vi "3030-HS - DAC.VI"() -> ()   [LabVIEW 2015]
uses:
  board.vis/Globals.vi
  <vilib>/Analysis/NI_AALBase.lvlib
panel:
  in  "extTrig":bool
  in  "ext. trig. slope":enum32{"1", "2", "3"}(radio)
  in  "send all":bool
  in  "Offset ADC 8":u16=49000
  in  "Offset ADC 3":u16=49000
  in  "Offset ADC 7":u16=49000
  in  "Offset ADC 2":u16=49000
  in  "Offset ADC 6":u16=49000
  in  "Offset ADC 1":u16=49000
  in  "Offset ADC 5":u16=49000
  in  "Offset ADC 4":u16=49000
  out "tRMS":dbl=11.563017373787728 format="%0#.1f"
  out "mean":dbl=8306.733333333334 format="%#_4f"
  in  "rms_pixel":u16=100
  in  "continuous":bool
  out "curr.block":u8=1
  out "Measure ON":bool
  in  "Board select\n1: board 1\n2: board 2\n3: both boards":u8=3
  in  "no.of blocks (nob)\npress enter":u32=1
  in  "block":u32(slide)=1 max=10 scale=0.9..1.0
  out "Signalverlaufgraph 2":u16[](graph)=[0, 0, 543, 543, 0, 1, 0, 0, 2, 2, 3, 3, 4, 4, 5, 5, 6, 6, 7, 7, 8, 8, 9, 9, 10, 10, 11, 11, 12, 12, 13, 13, 14, 14, 15, 15, 16, 16, 17, 17, 18, 18, 19, 19, 20, 20, 21, 21, 22, 22, 23, 23, 24, 24, 25, 25, 26, 26, 27, 27, 28, 28, 29, 29, 30, 30, 31, 31, 32, 32, 33, 33, 34, 34, 35, 35, 36, 36, 37, 37, 38, 38, 39, 39, 40, 40, 41, 41, 42, 42, 43, 43, 44, 44, 45, 45, 46, 46, 47, 47, 48, 48, 49, 49, 50, 50, 51, 51, 52, 52, 53, 53, 54, 54, 55, 55, 56, 56, 57, 57, 58, 58, 59, 59, 60, 60, 61, 61, 62, 62, 63, 63, 64, 64, 65, 65, 66, 66, 67, 67, 68, 68, 69, 69, 70, 70, 71, 71, 72, 72, 73, 73, 74, 74, 75, 75, 76, 76, 77, 77, 78, 78, 79, 79, 80, 80, 81, 81, 82, 82, 83, 83, 84, 84, 85, 85, 86, 86, 87, 87, 88, 88, 89, 89, 90, 90, 91, 91, 92, 92, 93, 93, 94, 94, 95, 95, 96, 96, 97, 97, 98, 98, 99, 99, 100, 100, 101, 101, 102, 102, 103, 103, 104, 104, 105, 105, 106, 106, 107, 107, 108, 108, 109, 109, 110, 110, 111, 111, 112, 112, 113, 113, 114, 114, 115, 115, 116, 116, 117, 117, 118, 118, 119, 119, 120, 120, 121, 121, 122, 122, 123, 123, 124, 124, 125, 125, 126, 126, 127, 127, 128, 128, 129, 129, 130, 130, 131, 131, 132, 132, 133, 133, 134, 134, 135, 135, 136, 136, 137, 137, 138, 138, 139, 139, 140, 140, 141, 141, 142, 142, 143, 143, 144, 144, 145, 145, 146, 146, 147, 147, 148, 148, 149, 149, 150, 150, 151, 151, 152, 152, 153, 153, 154, 154, 155, 155, 156, 156, 157, 157, 158, 158, 159, 159, 160, 160, 161, 161, 162, 162, 163, 163, 164, 164, 165, 165, 166, 166, 167, 167, 168, 168, 169, 169, 170, 170, 171, 171, 172, 172, 173, 173, 174, 174, 175, 175, 176, 176, 177, 177, 178, 178, 179, 179, 180, 180, 181, 181, 182, 182, 183, 183, 184, 184, 185, 185, 186, 186, 187, 187, 188, 188, 189, 189, 190, 190, 191, 191, 192, 192, 193, 193, 194, 194, 195, 195, 196, 196, 197, 197, 198, 198, 199, 199, 200, 200, 201, 201, 202, 202, 203, 203, 204, 204, 205, 205, 206, 206, 207, 207, 208, 208, 209, 209, 210, 210, 211, 211, 212, 212, 213, 213, 214, 214, 215, 215, 216, 216, 217, 217, 218, 218, 219, 219, 220, 220, 221, 221, 222, 222, 223, 223, 224, 224, 225, 225, 226, 226, 227, 227, 228, 228, 229, 229, 230, 230, 231, 231, 232, 232, 233, 233, 234, 234, 235, 235, 236, 236, 237, 237, 238, 238, 239, 239, 240, 240, 241, 241, 242, 242, 243, 243, 244, 244, 245, 245, 246, 246, 247, 247, 248, 248, 249, 249, 250, 250, 251, 251, 252, 252, 253, 253, 254, 254, 255, 255, 256, 256, 257, 257, 258, 258, 259, 259, 260, 260, 261, 261, 262, 262, 263, 263, 264, 264, 265, 265, 266, 266, 267, 267, 268, 268, 269, 269, 270, 270, 271, 271, 272, 272, 273, 273, 274, 274, 275, 275, 276, 276, 277, 277, 278, 278, 279, 279, 280, 280, 281, 281, 282, 282, 283, 283, 284, 284, 285, 285, 286, 286, 287, 287, 288, 288, 289, 289, 290, 290, 291, 291, 292, 292, 293, 293, 294, 294, 295, 295, 296, 296, 297, 297, 298, 298, 299, 299, 300, 300, 301, 301, 302, 302, 303, 303, 304, 304, 305, 305, 306, 306, 307, 307, 308, 308, 309, 309, 310, 310, 311, 311, 312, 312, 313, 313, 314, 314, 315, 315, 316, 316, 317, 317, 318, 318, 319, 319, 320, 320, 321, 321, 322, 322, 323, 323, 324, 324, 325, 325, 326, 326, 327, 327, 328, 328, 329, 329, 330, 330, 331, 331, 332, 332, 333, 333, 334, 334, 335, 335, 336, 336, 337, 337, 338, 338, 339, 339, 340, 340, 341, 341, 342, 342, 343, 343, 344, 344, 345, 345, 346, 346, 347, 347, 348, 348, 349, 349, 350, 350, 351, 351, 352, 352, 353, 353, 354, 354, 355, 355, 356, 356, 357, 357, 358, 358, 359, 359, 360, 360, 361, 361, 362, 362, 363, 363, 364, 364, 365, 365, 366, 366, 367, 367, 368, 368, 369, 369, 370, 370, 371, 371, 372, 372, 373, 373, 374, 374, 375, 375, 376, 376, 377, 377, 378, 378, 379, 379, 380, 380, 381, 381, 382, 382, 383, 383, 384, 384, 385, 385, 386, 386, 387, 387, 388, 388, 389, 389, 390, 390, 391, 391, 392, 392, 393, 393, 394, 394, 395, 395, 396, 396, 397, 397, 398, 398, 399, 399, 400, 400, 401, 401, 402, 402, 403, 403, 404, 404, 405, 405, 406, 406, 407, 407, 408, 408, 409, 409, 410, 410, 411, 411, 412, 412, 413, 413, 414, 414, 415, 415, 416, 416, 417, 417, 418, 418, 419, 419, 420, 420, 421, 421, 422, 422, 423, 423, 424, 424, 425, 425, 426, 426, 427, 427, 428, 428, 429, 429, 430, 430, 431, 431, 432, 432, 433, 433, 434, 434, 435, 435, 436, 436, 437, 437, 438, 438, 439, 439, 440, 440, 441, 441, 442, 442, 443, 443, 444, 444, 445, 445, 446, 446, 447, 447, 448, 448, 449, 449, 450, 450, 451, 451, 452, 452, 453, 453, 454, 454, 455, 455, 456, 456, 457, 457, 458, 458, 459, 459, 460, 460, 461, 461, 462, 462, 463, 463, 464, 464, 465, 465, 466, 466, 467, 467, 468, 468, 469, 469, 470, 470, 471, 471, 472, 472, 473, 473, 474, 474, 475, 475, 476, 476, 477, 477, 478, 478, 479, 479, 480, 480, 481, 481, 482, 482, 483, 483, 484, 484, 485, 485, 486, 486, 487, 487, 488, 488, 489, 489, 490, 490, 491, 491, 492, 492, 493, 493, 494, 494, 495, 495, 496, 496, 497, 497, 498, 498, 499, 499, 500, 500, 501, 501, 502, 502, 503, 503, 504, 504, 505, 505, 506, 506, 507, 507, 508, 508, 509, 509, 510, 510, 511, 511, 512, 512, 513, 513, 514, 514, 515, 515, 516, 516, 517, 517, 518, 518, 519, 519, 520, 520, 521, 521, 522, 522, 523, 523, 524, 524, 525, 525, 526, 526, 527, 527, 528, 528, 529, 529, 530, 530, 531, 531, 532, 532, 533, 533, 534, 534, 535, 535, 536, 536, 537, 537, 538, 538, 539, 539, 540, 540, 541, 541]
  out "Signalverlaufgraph":u16[](graph)=[8087, 8087, 8087, 8087, 49152, 1, 0, 50, 7170, 7170, 7521, 7730, 7840, 7916, 7976, 8049, 8112, 8160, 8204, 8214, 8236, 8264, 8286, 8290, 8324, 8328, 8343, 8353, 8359, 8375, 8388, 8394, 8403, 8403, 8394, 8394, 8388, 8378, 8378, 8372, 8362, 8347, 8340, 8334, 8331, 8343, 8340, 8331, 8321, 8312, 8309, 8312, 8302, 8315, 8321, 8324, 8328, 8312, 8309, 8299, 8312, 8305, 8309, 8293, 8318, 8309, 8305, 8315, 8321, 8318, 8312, 8305, 8312, 8290, 8302, 8274, 8280, 8290, 8305, 8305, 8299, 8324, 8305, 8302, 8302, 8302, 8312, 8309, 8315, 8309, 8296, 8296, 8299, 8305, 8312, 8309, 8299, 8302, 8305, 8296, 8305, 8299, 8299, 8296, 8293, 8302, 8280, 8290, 8302, 8305, 8286, 8283, 8283, 8280, 8293, 8290, 8290, 8274, 8280, 8271, 8252, 8258, 8245, 8255, 8248, 8258, 8264, 8271, 8286, 8283, 8277, 8280, 8274, 8264, 8258, 8261, 8255, 8255, 7094, 7258, 7407, 7568, 7742, 7900, 8005, 8103, 8135, 8157, 8198, 8207, 8245, 8252, 8264, 8271, 8286, 8296, 8318, 8343, 8340, 8343, 8334, 8334, 8315, 8340, 8334, 8328, 8324, 8318, 8309, 8302, 8290, 8286, 8290, 8283, 8267, 8255, 8264, 8255, 8252, 8255, 8242, 8264, 8258, 8258, 8248, 8248, 8264, 8236, 8229, 8255, 8248, 8245, 8255, 8267, 8258, 8248, 8264, 8248, 8236, 8226, 8217, 8245, 8226, 8233, 8236, 8239, 8252, 8252, 8261, 8245, 8267, 8258, 8258, 8258, 8252, 8255, 8258, 8239, 8239, 8242, 8239, 8239, 8226, 8236, 8233, 8239, 8214, 8226, 8223, 8226, 8226, 8242, 8229, 8229, 8242, 8229, 8233, 8220, 8226, 8220, 8226, 8226, 8229, 8229, 8226, 8201, 8198, 8207, 8204, 8192, 8192, 8201, 8220, 8229, 8214, 8214, 8226, 8229, 8233, 8214, 8214, 8198, 8201, 8198, 8201, 8201, 7535, 7706, 7869, 8014, 8163, 8298, 8426, 8504, 8546, 8599, 8642, 8670, 8685, 8716, 8734, 8738, 8745, 8777, 8787, 8816, 8833, 8833, 8841, 8855, 8830, 8833, 8823, 8816, 8805, 8805, 8798, 8787, 8787, 8773, 8791, 8787, 8777, 8773, 8773, 8766, 8759, 8759, 8763, 8763, 8766, 8763, 8752, 8755, 8741, 8748, 8745, 8734, 8741, 8755, 8763, 8763, 8763, 8755, 8745, 8745, 8734, 8755, 8745, 8748, 8724, 8724, 8731, 8745, 8741, 8741, 8745, 8731, 8738, 8741, 8738, 8741, 8731, 8745, 8748, 8748, 8731, 8731, 8727, 8713, 8720, 8731, 8727, 8731, 8720, 8724, 8724, 8731, 8716, 8731, 8734, 8731, 8741, 8734, 8724, 8716, 8709, 8724, 8720, 8709, 8713, 8706, 8713, 8695, 8706, 8695, 8692, 8688, 8685, 8688, 8685, 8706, 8695, 8699, 8709, 8702, 8702, 8706, 8702, 8692, 8699, 8695, 8688, 8688, 7100, 7287, 7448, 7622, 7783, 7942, 8049, 8125, 8160, 8204, 8233, 8239, 8271, 8283, 8286, 8302, 8312, 8312, 8328, 8350, 8359, 8381, 8356, 8350, 8350, 8350, 8334, 8321, 8328, 8334, 8318, 8321, 8309, 8296, 8293, 8293, 8305, 8286, 8277, 8280, 8277, 8283, 8280, 8283, 8290, 8280, 8274, 8264, 8258, 8277, 8258, 8274, 8271, 8280, 8283, 8302, 8283, 8290, 8293, 8280, 8258, 8274, 8264, 8271, 8271, 8271, 8271, 8290, 8277, 8267, 8283, 8267, 8267, 8264, 8286, 8283, 8280, 8290, 8286, 8290, 8283, 8274, 8290, 8271, 8277, 8274, 8286, 8274, 8261, 8261, 8261, 8267, 8274, 8274, 8274, 8283, 8280, 8261, 8264, 8267, 8261, 8258, 8258, 8248, 8248, 8245, 8239, 8236, 8226, 8233, 8239, 8223, 8223, 8226, 8245, 8239, 8245, 8255, 8245, 8255, 8255, 8236, 8245, 8236, 8239, 8229, 8245, 8245, 7777, 7964, 8135, 8271, 8435, 8546, 8647, 8717, 8783, 8834, 8856, 8872, 8878, 8888, 8900, 8922, 8919, 8938, 8954, 8967, 8979, 8992, 8986, 8992, 8967, 8986, 8964, 8957, 8941, 8945, 8941, 8941, 8941, 8932, 8935, 8922, 8926, 8926, 8926, 8922, 8919, 8907, 8910, 8919, 8907, 8922, 8913, 8919, 8907, 8900, 8903, 8897, 8903, 8903, 8922, 8919, 8922, 8913, 8916, 8910, 8903, 8891, 8888, 8891, 8869, 8891, 8891, 8907, 8910, 8888, 8903, 8916, 8900, 8903, 8916, 8910, 8913, 8897, 8913, 8894, 8897, 8897, 8884, 8894, 8888, 8891, 8891, 8891, 8894, 8884, 8884, 8888, 8878, 8884, 8897, 8888, 8881, 8888, 8884, 8897, 8875, 8884, 8881, 8894, 8891, 8884, 8865, 8853, 8853, 8850, 8862, 8840, 8853, 8853, 8869, 8859, 8853, 8865, 8872, 8894, 8881, 8862, 8856, 8853, 8853, 8865, 8862, 8862, 7511, 7713, 7894, 8089, 8284, 8458, 8603, 8702, 8773, 8794, 8830, 8851, 8865, 8876, 8890, 8873, 8894, 8915, 8919, 8968, 8982, 8968, 8979, 8968, 8954, 8968, 8940, 8936, 8940, 8929, 8922, 8929, 8901, 8901, 8915, 8912, 8897, 8912, 8897, 8897, 8887, 8876, 8873, 8869, 8897, 8897, 8883, 8883, 8862, 8876, 8851, 8869, 8876, 8876, 8894, 8897, 8876, 8890, 8883, 8880, 8851, 8858, 8841, 8841, 8830, 8844, 8862, 8880, 8873, 8876, 8887, 8883, 8876, 8887, 8890, 8890, 8887, 8897, 8901, 8890, 8876, 8851, 8883, 8862, 8851, 8873, 8876, 8869, 8855, 8862, 8851, 8855, 8851, 8858, 8876, 8869, 8865, 8869, 8858, 8865, 8862, 8873, 8844, 8862, 8858, 8869, 8855, 8844, 8837, 8841, 8837, 8826, 8823, 8837, 8848, 8862, 8844, 8865, 8862, 8855, 8862, 8844, 8830, 8830, 8826, 8830, 8844, 8844, 8071, 8252, 8397, 8555, 8714, 8853, 8960, 9027, 9071, 9115, 9138, 9150, 9191, 9195, 9210, 9204, 9217, 9229, 9245, 9264, 9293, 9280, 9283, 9277, 9264, 9277, 9248, 9245, 9242, 9232, 9229, 9229, 9236, 9210, 9223, 9220, 9226, 9204, 9195, 9201, 9195, 9204, 9191, 9188, 9207, 9204, 9198, 9204, 9195, 9176, 9188, 9176, 9179, 9198, 9188, 9182, 9179, 9198, 9195, 9188, 9179, 9179, 9166, 9169, 9163, 9157, 9172, 9188, 9179, 9191, 9188, 9182, 9188, 9201, 9188, 9198, 9179, 9188, 9191, 9188, 9179, 9188, 9176, 9182, 9179, 9185, 9182, 9179, 9169, 9157, 9163, 9169, 9172, 9182, 9201, 9191, 9185, 9188, 9182, 9169, 9172, 9172, 9163, 9176, 9179, 9169, 9153, 9157, 9141, 9150, 9147, 9131, 9122, 9160, 9153, 9160, 9160, 9153, 9160, 9163, 9157, 9157, 9134, 9138, 9147, 9125, 9144, 9144, 7606, 7787, 7957, 8122, 8299, 8432, 8543, 8603, 8657, 8682, 8720, 8742, 8761, 8767, 8780, 8783, 8796, 8799, 8808, 8818, 8837, 8843, 8853, 8834, 8827, 8837, 8812, 8802, 8802, 8799, 8780, 8790, 8767, 8771, 8796, 8790, 8771, 8767, 8764, 8764, 8752, 8742, 8755, 8764, 8767, 8783, 8755, 8752, 8739, 8742, 8755, 8739, 8748, 8736, 8761, 8764, 8758, 8767, 8758, 8761, 8742, 8736, 8736, 8736, 8698, 8704, 8736, 8736, 8748, 8748, 8764, 8761, 8755, 8758, 8745, 8748, 8755, 8758, 8755, 8758, 8739, 8736, 8723, 8729, 8726, 8736, 8736, 8739, 8733, 8717, 8714, 8720, 8710, 8729, 8752, 8742, 8745, 8739, 8739, 8742, 8726, 8733, 8742, 8739, 8736, 8729, 8707, 8707, 8704, 8717, 8704, 8695, 8688, 8695, 8723, 8729, 8720, 8717, 8720, 8739, 8733, 8707, 8710, 8710, 8704, 8717, 8742, 8742, 8264, 8226, 8188, 8141, 8097, 8097, 8097, 8097, 8097, 8097, 8097, 8097, 8097, 8097, 8097, 8097, 8097, 8097, 8097, 8097, 8097, 8097, 8097, 8097, 8097, 8097, 8097, 8097, 8097, 8097, 8097, 8097, 8097, 8097, 8097, 8097, 8097, 8097, 8097, 8097, 8097, 8097, 8097, 8097, 8097, 8097, 8097, 8097, 8097, 8097, 8097, 8097, 8097, 8097]
  out "boards recognised":u8=2
  in  "alloc mem":bool
  out "FREE \nRAM MB":dbl=13718.2421875
  out "BUILT-IN\nRAM MB":dbl=16271.7421875
  out "SEC":dbl=0.01
  out "MB RAM":dbl=0.20751953125
  in  "DAT in 10ns":u32
  in  "stop all":bool
  in  "start":bool
  in  "sample":u32(slide)=51 max=3000 scale=0.9..100.0
  in  "no.of samples (nos)":u32=1000
  in  "exposuretime[ms]":dbl=0.04 format="%.3f"
  # "press Esc to stop\nmeasurement"
  # "exit here"
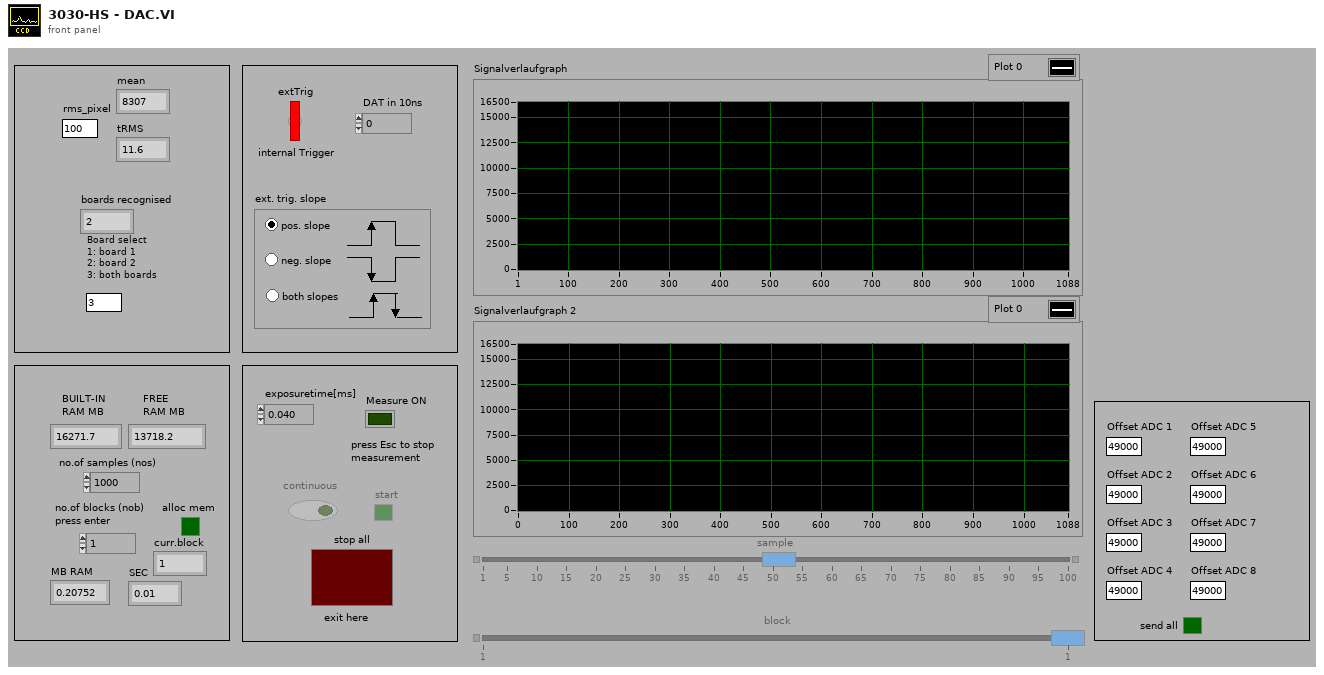
[diagram p1: front panel]
types:
  T1 = enum8{"Enabled", "Disabled", "Disabled and Grayed Out"}
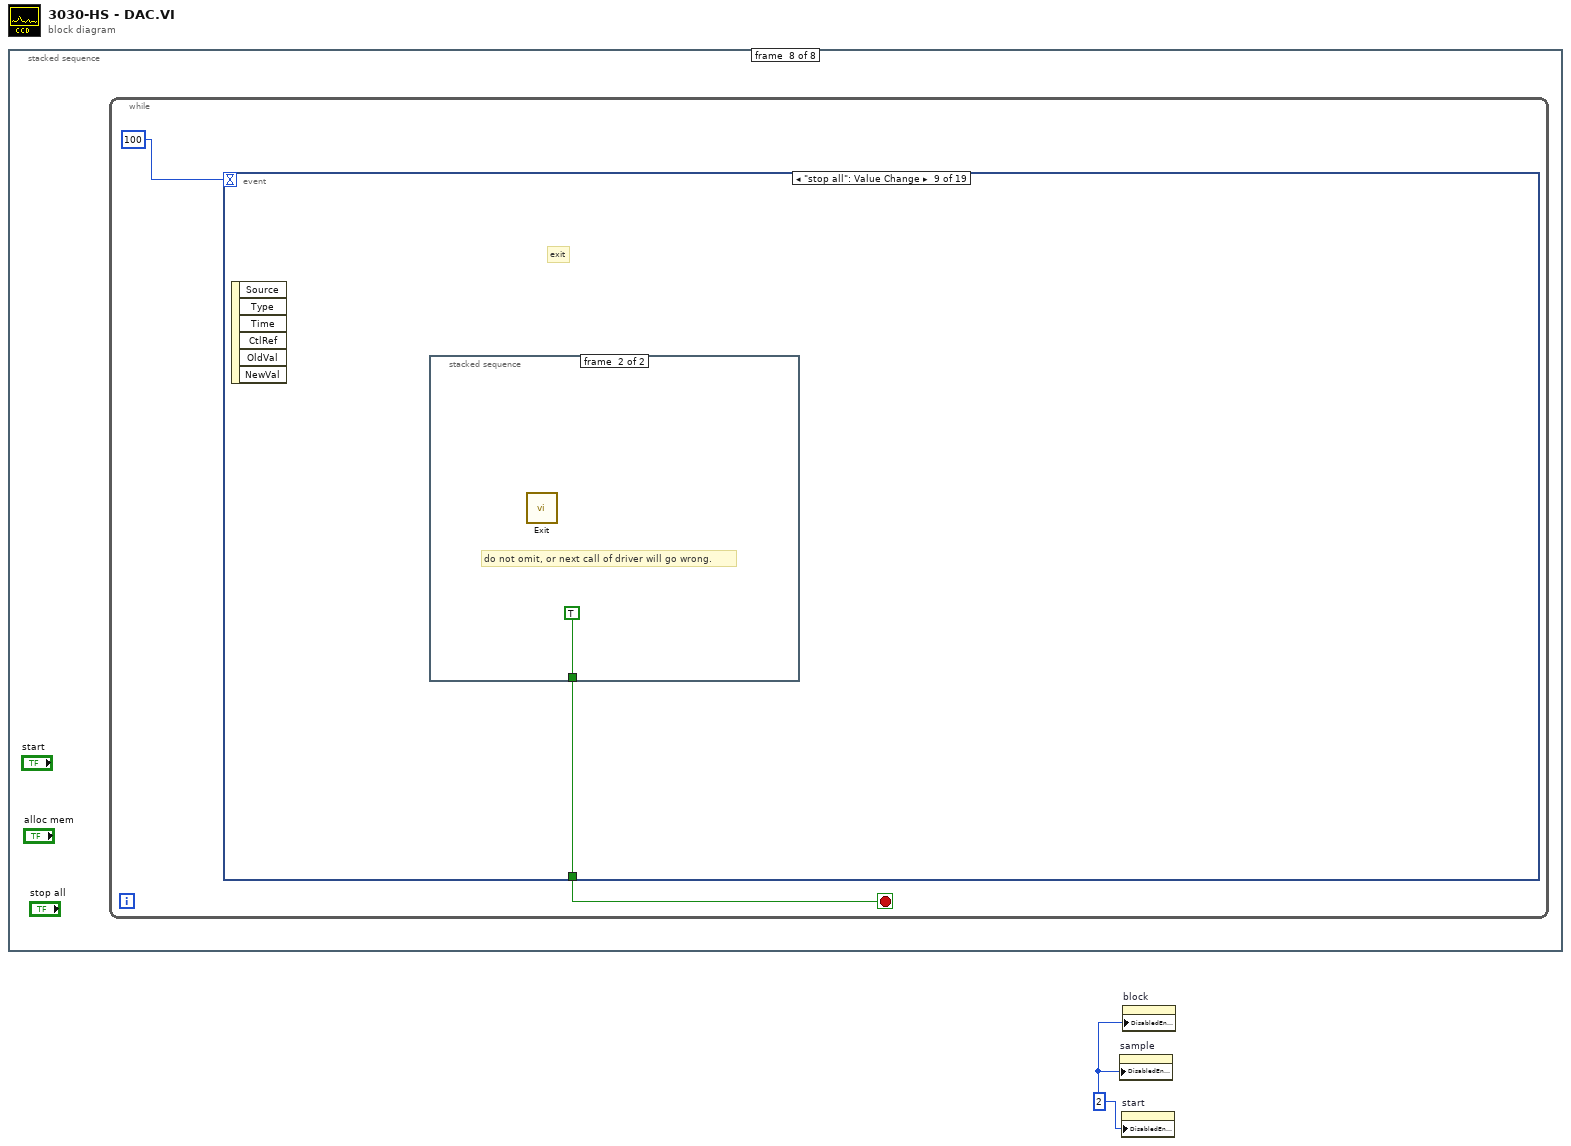
[diagram p0: block diagram]
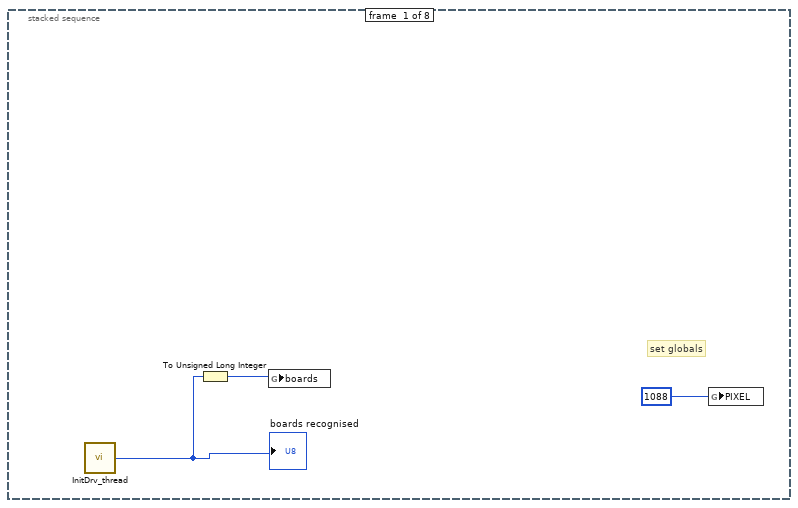
[diagram p2: hidden frame]
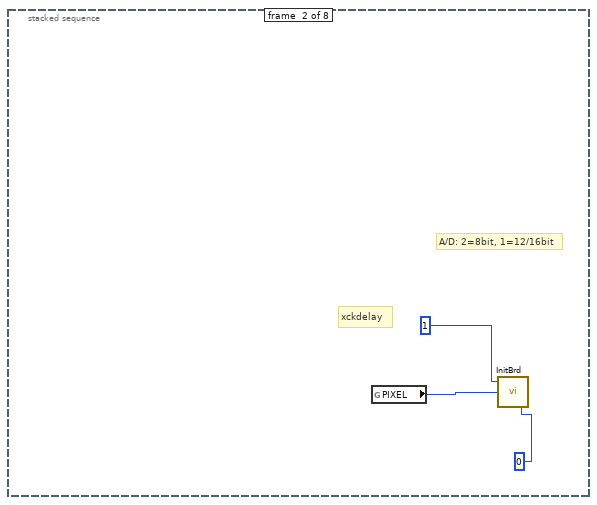
[diagram p3: hidden frame]
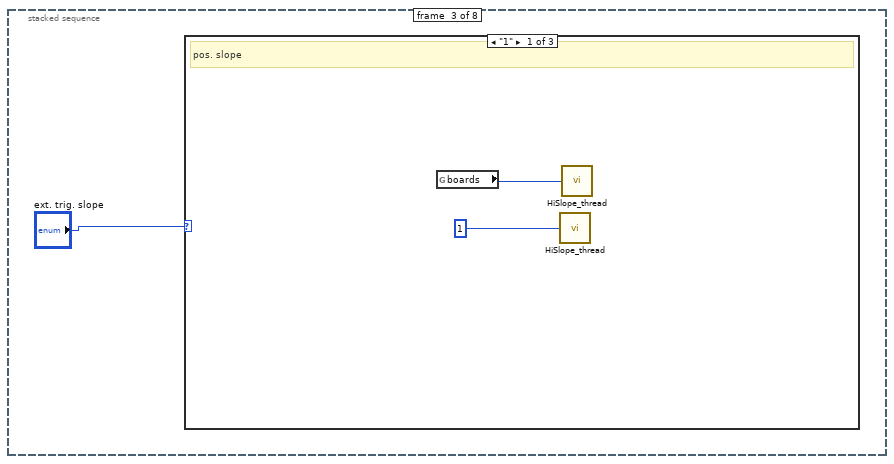
[diagram p4: hidden frame]
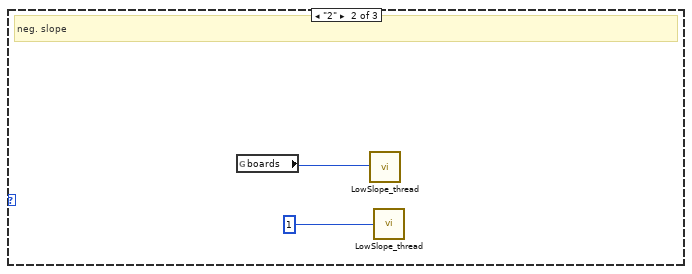
[diagram p5: hidden frame]
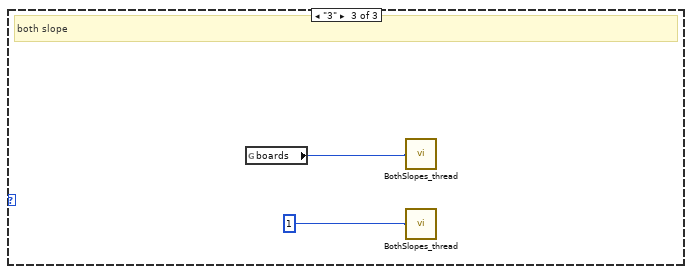
[diagram p6: hidden frame]
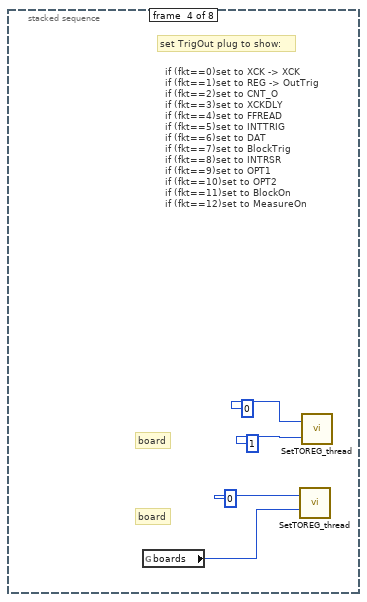
[diagram p7: hidden frame]
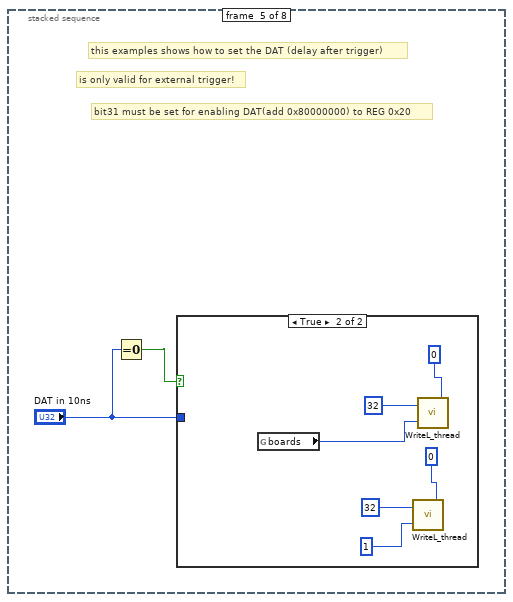
[diagram p8: hidden frame]
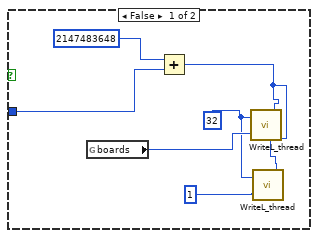
[diagram p9: hidden frame]
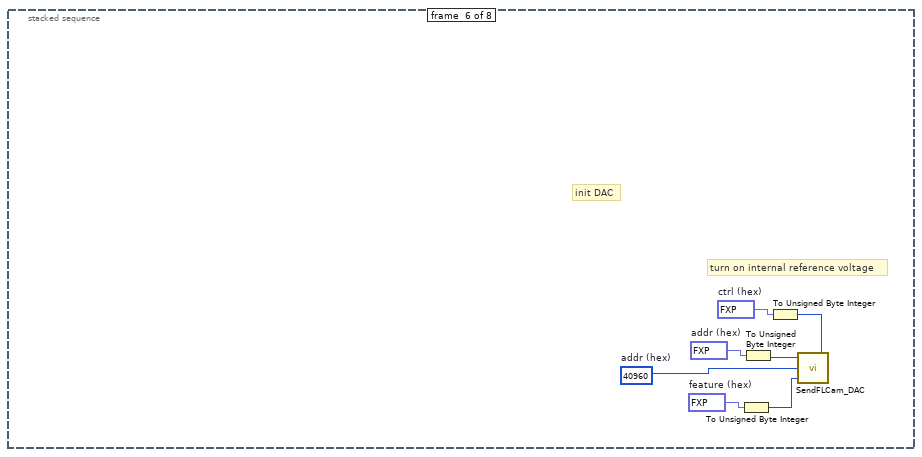
[diagram p10: hidden frame]
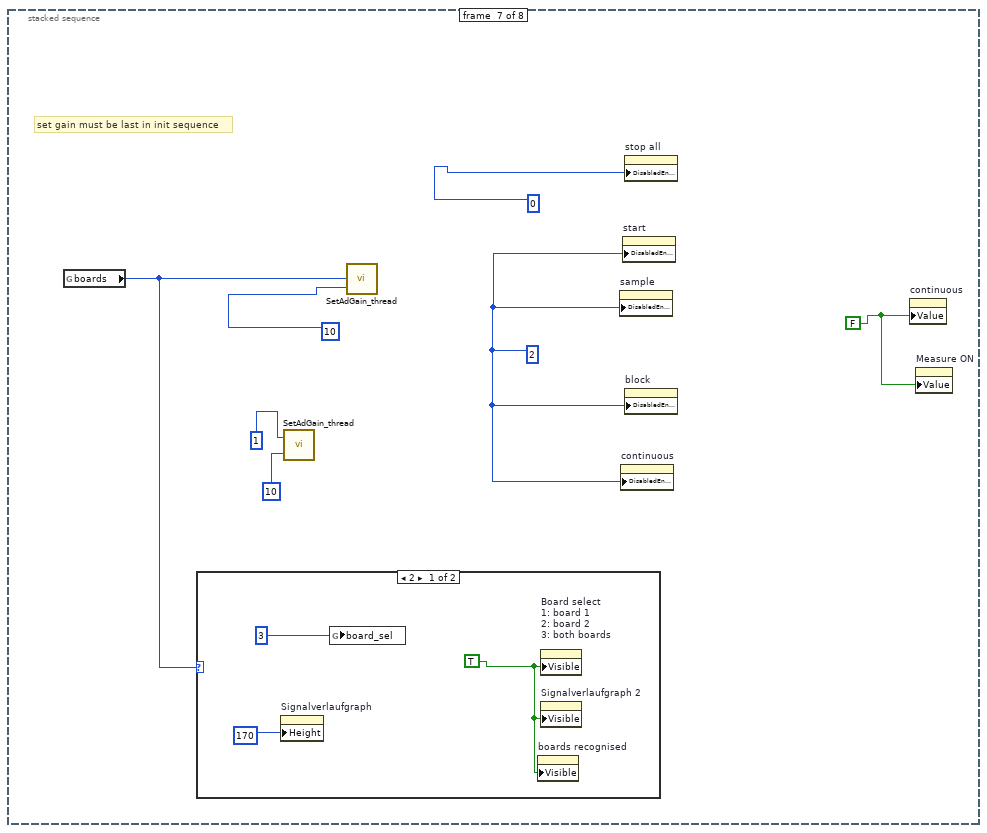
[diagram p11: hidden frame]
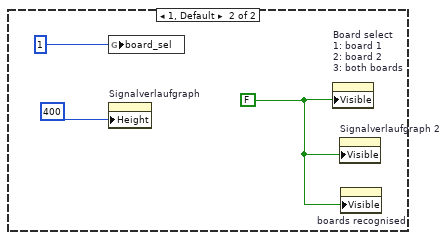
[diagram p12: hidden frame]
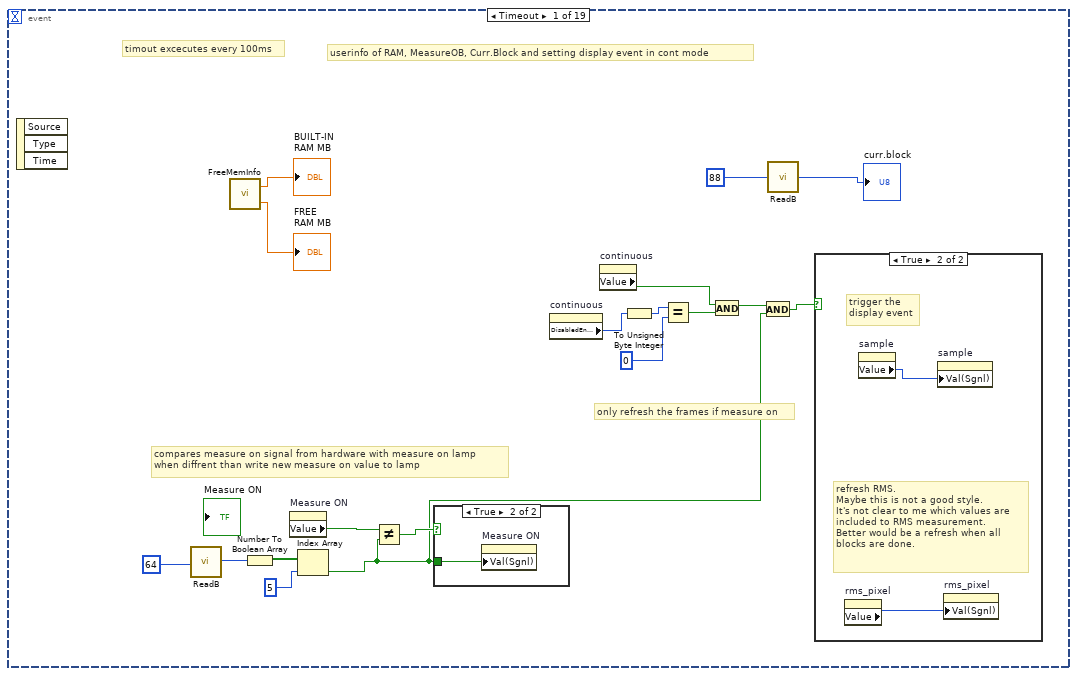
[diagram p13: hidden frame]
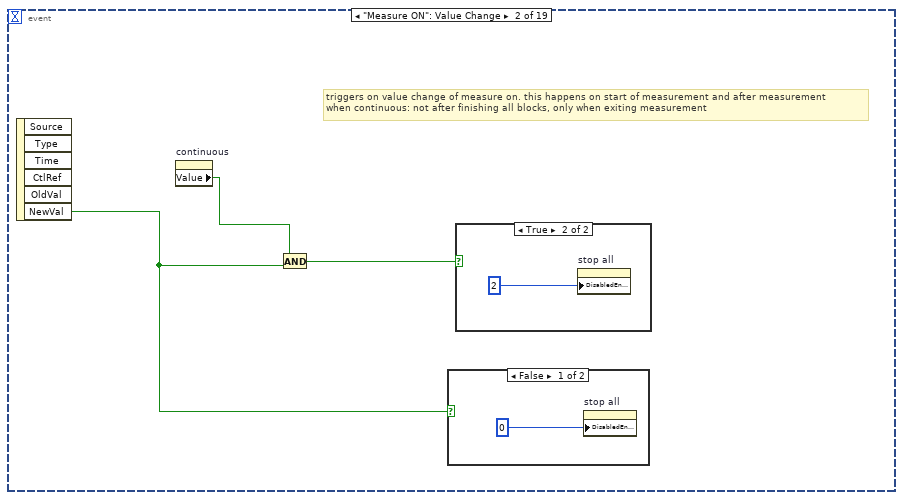
[diagram p16: hidden frame]
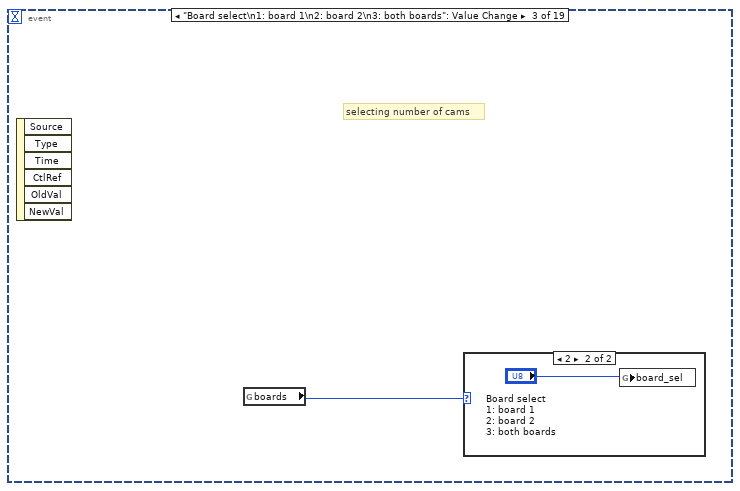
[diagram p19: hidden frame]
diagram:
  w1 = 2
  n1 = stacked-sequence {
    frame #0 {
      # "set globals"
      n2 = call "InitDrv_thread.vi"() -> ("Boards"=w2:u8)  [unwired: 1 in]
      "boards recognised" <- w2
      n3 = To Unsigned Long Integer(number=w2) -> (unsigned 32bit integer=w3:u32)
      n4 = global write "Globals.vi" "boards"(w3) -> ()
      n5 = global write "Globals.vi" "PIXEL"(u32 1088) -> ()
    }
    frame #1 {
      # "xckdelay"
      # "A/D: 2=8bit, 1=12/16bit"
      n6 = global read "Globals.vi" "PIXEL"() -> (w7:u32)
      n7 = call "InitBrd.vi"("xckdly"=u32 0, "pixel"=w7, "flag816"=u32 1) -> ()  [unwired: 3 in]
    }
    frame #2 {
      n8 = case shown="\"1\"" "ext. trig. slope" {
        frame "1" {
          # "pos. slope"
          n9 = global read "Globals.vi" "boards"() -> (w9:u32)
          n10 = call "HiSlope_thread.vi"("board"=u32 1) -> ()  [unwired: 1 in]
          n11 = call "HiSlope_thread.vi"("board"=w9) -> ()  [unwired: 1 in]
        }
        frame "2" {
          # "neg. slope"
          n12 = global read "Globals.vi" "boards"() -> (w12:u32)
          n13 = call "LowSlope_thread.vi"("board"=w12) -> ()  [unwired: 1 in]
          n14 = call "LowSlope_thread.vi"("board"=u32 1) -> ()  [unwired: 1 in]
        }
        frame "3" {
          # "both slope"
          n15 = global read "Globals.vi" "boards"() -> (w13:u32)
          n16 = call "BothSlopes_thread.vi"("board"=w13) -> ()  [unwired: 1 in]
          n17 = call "BothSlopes_thread.vi"("board"=u32 1) -> ()  [unwired: 1 in]
        }
      }
    }
    frame #3 {
      # "board"
      # "board"
      # "set TrigOut plug to show:"
      # "if (fkt==0)set to XCK -> XCK\nif (fkt==1)set to REG -> OutTrig\nif (fkt==2)set to CNT_O\nif (fkt==3)set to XCKDLY\nif (fkt==4)set to FFREAD\nif (fkt==5)set to INTTRIG\nif (fkt==6)set to DAT\nif (fkt==7)set to BlockTrig\nif (fkt==8)set to INTRSR\nif (fkt==9)set to OPT1\nif (fkt==10)set to OPT2\nif (fkt==11)set to BlockOn\nif (fkt==12)set to MeasureOn"
      n18 = global read "Globals.vi" "boards"() -> (w18:u32)
      n19 = call "SetTOREG_thread.vi"("board"=w18, "fkt"=u8 0) -> ()  [unwired: 1 in]
      n20 = call "SetTOREG_thread.vi"("board"=u32 1, "fkt"=u8 0) -> ()  [unwired: 1 in]
    }
    frame #4 {
      # "bit31 must be set for enabling DAT(add 0x80000000) to REG 0x20"
      # "is only valid for external trigger!"
      # "this examples shows how to set the DAT (delay after trigger)"
      n21 = Equal To 0?(x="DAT in 10ns") -> (x = 0?=w20:bool)
      n22 = case shown="True" w20 {
        tunnel: "DAT in 10ns" -> [w25 _]
        frame False {
          w22 = u32 32
          n23 = global read "Globals.vi" "boards"() -> (w24:u32)
          n24 = Add(x=u32 2147483648, y=w25) -> (x+y=w23:u32)
          n25 = call "WriteL_thread.vi"("val"=w23, "board"=w24, "offset"=w22) -> ()
          n26 = call "WriteL_thread.vi"("val"=w23, "board"=u32 1, "offset"=w22) -> ()
        }
        frame True {
          n27 = global read "Globals.vi" "boards"() -> (w31:u32)
          n28 = call "WriteL_thread.vi"("val"=u32 0, "board"=u32 1, "offset"=u32 32) -> ()
          n29 = call "WriteL_thread.vi"("val"=u32 0, "board"=w31, "offset"=u32 32) -> ()
        }
      }
    }
    frame #5 {
      w33 = u16 40960  # addr (hex)
      w36 = fxp<+,4,4> 0.0  # feature (hex)
      w37 = fxp<+,4,4> 0.0  # addr (hex)
      w39 = fxp<+,4,4> 9.0  # ctrl (hex)
      # "turn on internal reference voltage"
      # "init DAC"
      n30 = To Unsigned Byte Integer(number=w36) -> (unsigned 8bit integer=w35:u8)
      n31 = To Unsigned Byte Integer(number=w37) -> (unsigned 8bit integer=w34:u8)
      n32 = To Unsigned Byte Integer(number=w39) -> (unsigned 8bit integer=w38:u8)
      n33 = call "SendFLCam_DAC.vi"("ctrl"=w38, "feature"=w35, "data"=w33, "addr"=w34) -> ()
    }
    frame #6 {
      w40 = FALSE
      w46 = 2
      # "set gain must be last in init sequence"
      n34 = global read "Globals.vi" "boards"() -> (w44:u32)
      n35 = case shown="2" w44 {
        frame 2 {
          w49 = TRUE
          n36 = property on="Signalverlaufgraph" class="WFGraph (strict)"("Height"=u8 170) -> ()  [unwired: 2 in, 2 out]
          n37 = global write "Globals.vi" "board_sel"(u8 3) -> ()
          n38 = property on="boards recognised" class="DigNum (strict)"("Visible"=w49) -> ()  [unwired: 2 in, 2 out]
          n39 = property on="Board select\n1: board 1\n2: board 2\n3: both boards" class="DigNum (strict)"("Visible"=w49) -> ()  [unwired: 2 in, 2 out]
          n40 = property on="Signalverlaufgraph 2" class="WFGraph (strict)"("Visible"=w49) -> ()  [unwired: 2 in, 2 out]
        }
        frame 1, Default {
          w50 = FALSE
          n41 = global write "Globals.vi" "board_sel"(u8 1) -> ()
          n42 = property on="Signalverlaufgraph" class="WFGraph (strict)"("Height"=400) -> ()  [unwired: 2 in, 2 out]
          n43 = property on="Board select\n1: board 1\n2: board 2\n3: both boards" class="DigNum (strict)"("Visible"=w50) -> ()  [unwired: 2 in, 2 out]
          n44 = property on="Signalverlaufgraph 2" class="WFGraph (strict)"("Visible"=w50) -> ()  [unwired: 2 in, 2 out]
          n45 = property on="boards recognised" class="DigNum (strict)"("Visible"=w50) -> ()  [unwired: 2 in, 2 out]
        }
      }
      n46 = call "SetAdGain_thread.vi"("gain"=u8 10, "board"=u32 1) -> ()  [unwired: 1 in]
      n47 = call "SetAdGain_thread.vi"("gain"=u8 10, "board"=w44) -> ()  [unwired: 1 in]
      n48 = property on="sample" class="Slide (strict)"("DisabledEnum"=w46) -> ()  [unwired: 2 in, 2 out]
      n49 = property on="continuous" class="Bool (strict)"("DisabledEnum"=w46) -> ()  [unwired: 2 in, 2 out]
      n50 = property on="start" class="Bool (strict)"("DisabledEnum"=w46) -> ()  [unwired: 2 in, 2 out]
      n51 = property on="stop all" class="Bool (strict)"("DisabledEnum"=0) -> ()  [unwired: 2 in, 2 out]
      n52 = property on="block" class="Slide (strict)"("DisabledEnum"=w46) -> ()  [unwired: 2 in, 2 out]
      n53 = property on="continuous" class="Bool (strict)"("Value"=w40) -> ()  [unwired: 2 in, 2 out]
      n54 = property on="Measure ON" class="Bool (strict)"("Value"=w40) -> ()  [unwired: 2 in, 2 out]
    }
    frame #7 {
      n55 = while {
        stop <- w54 stop-if-true
        n56 = event shown="[8] \"stop all\": Value Change" {
          selector: _ -> [_ _ _ _ _ _ _ _ _ _ _ _ _ _ _ _ _ _ _]
          dyn-events: _ -> [_ _ _ _ _ _ _ _ _ _ _ _ _ _ _ _ _ _ _]
          timeout: 100 -> [_ _ _ _ _ _ _ _ _ _ _ _ _ _ _ _ _ _ _]
          tunnel: [_ _ _ _ _ _ _ _ w160 _ _ _ _ _ _ _ _ _ _] -> w54
          event Timeout {
            # "only refresh the frames if measure on"
            # "compares measure on signal from hardware with measure on lamp\nwhen diffrent than write new measure on value to lamp"
            # "timout excecutes every 100ms"
            # "userinfo of RAM, MeasureOB, Curr.Block and setting display event in cont mode"
            n57 = event-data() -> ()  [unwired: 1 in, 3 out]
            n58 = call "ReadB.vi"("Offset"=u32 64) -> ("Data"=w69:u8)
            n59 = call "FreeMemInfo.vi"() -> ("PhysicalSpace"=→"BUILT-IN\nRAM MB":dbl, "PhysicalFreeSpace"=→"FREE \nRAM MB":dbl)  [unwired: 1 in]
            n60 = Number To Boolean Array(number=w69) -> (Boolean array=w68:bool[])
            n61 = property on="Measure ON" class="Bool (strict)"() -> ("Value"=w62:bool)  [unwired: 2 in, 2 out]
            n62 = Index Array(array=w68, index=5) -> (element=w58:bool)
            n63 = Not Equal?(x=w62, y=w58) -> (x != y?=w61:bool)
            n64 = case shown="True" w61 {
              tunnel: w58 -> [_ w73]
              frame False {
              }
              frame True {
                n65 = property on="Measure ON" class="Bool (strict)"("Val(Sgnl)"=w73) -> ()  [unwired: 2 in, 2 out]
              }
            }
            n66 = property on="continuous" class="Bool (strict)"() -> ("DisabledEnum"=w55:T1)  [unwired: 2 in, 2 out]
            n67 = property on="continuous" class="Bool (strict)"() -> ("Value"=w64:bool)  [unwired: 2 in, 2 out]
            n68 = To Unsigned Byte Integer(number=w55) -> (unsigned 8bit integer=w56:u8)
            n69 = Equal?(x=w56, y=u8 0) -> (x = y?=w63:bool)
            n70 = And(x=w64, y=w63) -> (x .and. y?=w60:bool)
            n71 = And(x=w60, y=w58) -> (x .and. y?=w59:bool)
            n72 = call "ReadB.vi"("Offset"=u32 88) -> ("Data"=→"curr.block":u8)
            n73 = case shown="True" w59 {
              frame False {
              }
              frame True {
                # "refresh RMS.\nMaybe this is not a good style.\nIt's not clear to me which values are \nincluded to RMS measurement.\nBetter would be a refresh when all\nblocks are done."
                # "trigger the \ndisplay event"
                n74 = property on="rms_pixel" class="DigNum (strict)"() -> ("Value"=w74:u16)  [unwired: 2 in, 2 out]
                n75 = property on="sample" class="Slide (strict)"() -> ("Value"=w75:u32)  [unwired: 2 in, 2 out]
                n76 = property on="sample" class="Slide (strict)"("Val(Sgnl)"=w75) -> ()  [unwired: 2 in, 2 out]
                n77 = property on="rms_pixel" class="DigNum (strict)"("Val(Sgnl)"=w74) -> ()  [unwired: 2 in, 2 out]
              }
            }
          }
          event "Measure ON": Value Change {
            # "triggers on value change of measure on. this happens on start of measurement and after measurement\nwhen continuous: not after finishing all blocks, only when exiting measurement"
            n78 = event-data() -> ("NewVal"=w76:bool)  [unwired: 1 in, 5 out]
            n79 = property on="continuous" class="Bool (strict)"() -> ("Value"=w77:bool)  [unwired: 2 in, 2 out]
            n80 = And(x=w77, y=w76) -> (x .and. y?=w78:bool)
            n81 = case shown="False" w76 {
              frame False {
                n82 = property on="stop all" class="Bool (strict)"("DisabledEnum"=0) -> ()  [unwired: 2 in, 2 out]
              }
              frame True {
              }
            }
            n83 = case shown="True" w78 {
              frame False {
              }
              frame True {
                n84 = property on="stop all" class="Bool (strict)"("DisabledEnum"=2) -> ()  [unwired: 2 in, 2 out]
              }
            }
          }
          event "Board select\n1: board 1\n2: board 2\n3: both boards": Value Change {
            # "selecting number of cams"
            n85 = event-data() -> ()  [unwired: 1 in, 6 out]
            n86 = global read "Globals.vi" "boards"() -> (w81:u32)
            n87 = case shown="2" w81 {
              frame 0, Default {
              }
              frame 2 {
                n88 = global write "Globals.vi" "board_sel"("Board select\n1: board 1\n2: board 2\n3: both boards") -> ()
              }
            }
          }
          event "continuous": Value Change {
            # "setting continuos mode"
            n89 = event-data() -> ()  [unwired: 1 in, 6 out]
            n90 = case shown="False" "continuous" {
              tunnel: [u8 0 u8 1] -> w83
              frame False {
              }
              frame True {
              }
            }
            n91 = call "contFFLoop.vi"("Numeric"=w83) -> ()  [unwired: 1 in]
          }
          event "alloc mem": Value Change {
            w89 = 0
            # "update params"
            # "Setup DMA"
            n92 = event-data() -> ()  [unwired: 1 in, 6 out]
            n93 = global read "Globals.vi" "nob"() -> (w87:u32)
            n94 = global read "Globals.vi" "nos"() -> (w88:u32)
            n95 = global read "Globals.vi" "boards"() -> (w92:u32)
            n96 = case shown="2" w92 {
              selector: w92 -> [_ w93]
              tunnel: w88 -> [_ w94]
              tunnel: w87 -> [_ w95]
              frame 1, Default {
              }
              frame 2 {
                # "Setup DMA"
                n97 = call "SetupDMA_thread.vi"("blocks"=w95, "nos"=w94, "Drv"=w93) -> ()  [unwired: 2 in]
              }
            }
            n98 = call "SetupDMA_thread.vi"("blocks"=w87, "nos"=w88, "Drv"=u32 1) -> ()  [unwired: 2 in]
            n99 = property on="continuous" class="Bool (strict)"("DisabledEnum"=w89) -> ()  [unwired: 2 in, 2 out]
            n100 = property on="block" class="Slide (strict)"("DisabledEnum"=w89) -> ()  [unwired: 2 in, 2 out]
            n101 = property on="sample" class="Slide (strict)"("DisabledEnum"=w89) -> ()  [unwired: 2 in, 2 out]
            n102 = property on="exposuretime[ms]" class="DigNum (strict)"() -> ("Value"=w91:dbl)  [unwired: 2 in, 2 out]
            n103 = property on="start" class="Bool (strict)"("DisabledEnum"=w89) -> ()  [unwired: 2 in, 2 out]
            n104 = property on="exposuretime[ms]" class="DigNum (strict)"("Val(Sgnl)"=w91) -> ()  [unwired: 2 in, 2 out]
          }
          event "start": Mouse Down {
            # "start measurement"
            # "only 1st PCI board is used for ext. trig."
            # "ext. block trig\n0: internal: Space\n1: PCI \"I\"\n2: S1\n3: S2"
            # "block trigger 0/1\n0: internal -> next block is started immediately \n1: external -> each block has an own trigger"
            n105 = event-data() -> ()  [unwired: 1 in, 8 out]
            n106 = global read "Globals.vi" "exp time"() -> (w102:dbl)
            n107 = Multiply(x=1000.0, y=w102) -> (x*y=w104:dbl)
            n108 = global read "Globals.vi" "board_sel"() -> (w98:u8)
            n109 = To Unsigned Long Integer(number=w104) -> (unsigned 32bit integer=w100:u32)
            n110 = case shown="True" "extTrig" {
              tunnel: [u8 0 u8 1] -> w96
              frame False {
              }
              frame True {
              }
            }
            n111 = call "ReadFFLoop_thread.vi"("blocktrigger"=u8 0, "btrig_ch"=u8 0, "ExtTrig"=w96, "cam_sel"=w98, "exptus"=w100) -> ()  [unwired: 1 in]
          }
          event "sample", "block": Value Change {
            w118 = u32 1
            # "when selecting a value\nbigger than possible\nnos or nob, a dummy \nvalue \"1\" is chosen\n\nTODO:\ninsert error handling\nwith lower values than 1"
            # "display"
            n112 = event-data() -> ()  [unwired: 1 in, 6 out]
            n113 = global read "Globals.vi" "boards"() -> (w121:u32)
            n114 = global read "Globals.vi" "nob"() -> (w110:u32)
            n115 = global read "Globals.vi" "nos"() -> (w117:u32)
            n116 = Greater Or Equal?(x=w110, y="block") -> (x >= y?=w113:bool)
            n117 = Greater Or Equal?(x=w117, y="sample") -> (x >= y?=w116:bool)
            n118 = global read "Globals.vi" "PIXEL"() -> (w107:u32)
            n119 = case shown="False" w113 {
              tunnel: [u32 1 w126] -> w112
              tunnel: "block" -> [_ w126]
              frame False {
                n120 = call "Display Message to User"() -> ()  [unwired: 10 in, 2 out]
              }
              frame True {
              }
            }
            n121 = case shown="False" w116 {
              tunnel: [u32 1 w128] -> w115
              tunnel: "sample" -> [_ w128]
              frame False {
                n122 = call "Display Message to User2"() -> ()  [unwired: 10 in, 2 out]
              }
              frame True {
              }
            }
            n123 = To Long Integer(number=w107) -> (32bit integer=w108:i32)
            n124 = Initialize Array(u16 100, w108) -> (w124:u16[])
            n125 = Subtract(x=w115, y=w118) -> (x-y=w120:u32)
            n126 = Subtract(x=w112, y=w118) -> (x-y=w119:u32)
            n127 = case shown="2" w121 {
              selector: w121 -> [_ w133]
              tunnel: w120 -> [_ w134]
              tunnel: w119 -> [_ w131]
              frame 0, Default {
              }
              frame 2 {
                n128 = global read "Globals.vi" "PIXEL"() -> (w129:u32)
                n129 = To Long Integer(number=w129) -> (32bit integer=w130:i32)
                n130 = Initialize Array(u16 100, w130) -> (w136:u16[])
                n131 = call "ReturnFrame.vi"("Data Values In"=w136, "curr_nob"=w131, "curr_nos"=w134, "Drv"=w133) -> ("Data Values Out"=→"Signalverlaufgraph 2":u16[])  [unwired: 1 in]
              }
            }
            n132 = call "ReturnFrame.vi"("Data Values In"=w124, "curr_nob"=w119, "curr_nos"=w120, "Drv"=u32 1) -> ("Data Values Out"=→"Signalverlaufgraph":u16[])  [unwired: 1 in]
          }
          event "no.of samples (nos)", "no.of blocks (nob)\npress enter", "exposuretime[ms]": Value Change {
            # "calculation of MB RAM an SEC and setting scale max"
            # "MB"
            # "ushort"
            n133 = event-data() -> ()  [unwired: 1 in, 7 out]
            n134 = global read "Globals.vi" "PIXEL"() -> (w159:u32)
            n135 = Multiply(x="no.of samples (nos)", y=w159) -> (x*y=w157:u32)
            n136 = Multiply(x=w157, y=u32 2) -> (x*y=w137:u32)
            n137 = global read "Globals.vi" "boards"() -> (w158:u32)
            n138 = global read "Globals.vi" "nos"() -> (w141:u32)
            n139 = global read "Globals.vi" "nob"() -> (w139:u32)
            n140 = Multiply(x=w137, y=w158) -> (x*y=w147:u32)
            n141 = To Double Precision Float(number=w147) -> (double precision float=w146:dbl)
            n142 = To Double Precision Float(number=w141) -> (double precision float=w140:dbl)
            n143 = Divide(x=w146, y=1048576.0) -> (x/y=w149:dbl)
            n144 = To Double Precision Float(number=w139) -> (double precision float=w138:dbl)
            n145 = To Double Precision Float(number="no.of blocks (nob)\npress enter") -> (double precision float=w144:dbl)
            n146 = property on="sample" class="Slide (strict)"("Scale.Maximum"=w140) -> ()  [unwired: 2 in, 2 out]
            n147 = property on="block" class="Slide (strict)"("Scale.Maximum"=w138) -> ()  [unwired: 2 in, 2 out]
            n148 = Multiply(x=w149, y=w144) -> (x*y=→"MB RAM":dbl)
            n149 = global write "Globals.vi" "nos"("no.of samples (nos)") -> ()
            n150 = Multiply(x="no.of samples (nos)", y="no.of blocks (nob)\npress enter") -> (x*y=w142:u32)
            n151 = global write "Globals.vi" "nob"("no.of blocks (nob)\npress enter") -> ()
            n152 = To Double Precision Float(number=w142) -> (double precision float=w143:dbl)
            n153 = global write "Globals.vi" "exp time"("exposuretime[ms]") -> ()
            n154 = Multiply(x="exposuretime[ms]", y=w143) -> (x*y=w155:dbl)
            n155 = Divide(x=w155, y=1000.0) -> (x/y=→"SEC":dbl)
          }
          event "stop all": Value Change {
            # "exit"
            n156 = event-data() -> ()  [unwired: 1 in, 6 out]
            n157 = stacked-sequence {
              tunnel: [_ TRUE] -> w160
              frame #0 {
                n158 = call "FFStop.vi"() -> ()  [unwired: 1 in]
              }
              frame #1 {
                # "do not omit, or next call of driver will go wrong."
                n159 = call "Exit.vi"() -> ()  [unwired: 1 in]
              }
            }
          }
          event "rms_pixel": Value Change {
            # "one array with all values (except first 10)\nat index Pixel from all blocks"
            n160 = event-data() -> ()  [unwired: 1 in, 6 out]
            n161 = global read "Globals.vi" "nos"() -> (w166:u32)
            n162 = global read "Globals.vi" "nob"() -> (w167:u32)
            n163 = for {
              N: w167 -> [_]
              tunnel: w166 -> [w168]
              tunnel: [w170] -> w163 mode=concatenating
              i -> [w174]
              # "delete first 10 values"
              # "array of all values\nat index Pixel"
              n164 = To Long Integer(number=w168) -> (32bit integer=w169:i32)
              n165 = for {
                N: w169 -> [_]
                tunnel: w174 -> [w179]
                tunnel: [w183] -> w171 mode=indexing
                i -> [w181]
                # "use only value at index \"Pixel\""
                # "init array of size PIXEL\nwith value 100"
                n166 = global read "Globals.vi" "PIXEL"() -> (w175:u32)
                n167 = To Long Integer(number=w175) -> (32bit integer=w176:i32)
                n168 = To Unsigned Long Integer(number=w179) -> (unsigned 32bit integer=w180:u32)
                n169 = To Unsigned Long Integer(number=w181) -> (unsigned 32bit integer=w182:u32)
                n170 = Initialize Array(u16 100, w176) -> (w185:u16[])
                n171 = call "ReturnFrame.vi"("Data Values In"=w185, "curr_nob"=w180, "curr_nos"=w182, "Drv"=u32 1) -> ("Data Values Out"=w184:u16[])  [unwired: 1 in]
                n172 = To Long Integer(number="rms_pixel") -> (32bit integer=w177:i32)
                n173 = Index Array(array=w184, index=w177) -> (element=w183:u16)
              }
              n174 = Delete From Array(array=w171, length=10, index=0) -> (array with subset deleted=w170:u16[])  [unwired: 1 out]
            }
            n175 = To Double Precision Float(number=w163) -> (double precision float=w162:dbl[])
            n176 = call <vilib>:"Std Deviation and Variance.vi"("X"=w162) -> ("mean"=→"mean":dbl, "standard deviation"=→"tRMS":dbl)  [unwired: 1 in, 1 out]
          }
          event "Offset ADC 4": Value Change {
            w190 = fxp<+,4,4> 0.0  # feature (hex)
            w191 = fxp<+,4,4> 0.0  # addr (hex)
            w193 = fxp<+,4,4> 3.0  # ctrl (hex)
            # "Register CHA"
            # "ctrl: write and update DAC register"
            n177 = event-data() -> ()  [unwired: 1 in, 6 out]
            n178 = To Unsigned Byte Integer(number=w190) -> (unsigned 8bit integer=w189:u8)
            n179 = To Unsigned Byte Integer(number=w191) -> (unsigned 8bit integer=w188:u8)
            n180 = To Unsigned Byte Integer(number=w193) -> (unsigned 8bit integer=w192:u8)
            n181 = call "SendFLCam_DAC.vi"("ctrl"=w192, "feature"=w189, "data"="Offset ADC 4", "addr"=w188) -> ()
          }
          event "Offset ADC 5": Value Change {
            w198 = fxp<+,4,4> 0.0  # feature (hex)
            w199 = fxp<+,4,4> 1.0  # addr (hex)
            w201 = fxp<+,4,4> 3.0  # ctrl (hex)
            # "Register CHB"
            # "ctrl: write and update DAC register"
            n182 = event-data() -> ()  [unwired: 1 in, 6 out]
            n183 = To Unsigned Byte Integer(number=w198) -> (unsigned 8bit integer=w197:u8)
            n184 = To Unsigned Byte Integer(number=w199) -> (unsigned 8bit integer=w196:u8)
            n185 = To Unsigned Byte Integer(number=w201) -> (unsigned 8bit integer=w200:u8)
            n186 = call "SendFLCam_DAC.vi"("ctrl"=w200, "feature"=w197, "data"="Offset ADC 5", "addr"=w196) -> ()
          }
          event "Offset ADC 1": Value Change {
            w205 = fxp<+,4,4> 0.0  # feature (hex)
            w206 = fxp<+,4,4> 2.0  # addr (hex)
            w208 = fxp<+,4,4> 3.0  # ctrl (hex)
            # "Register CHC"
            # "ctrl: write and update DAC register"
            n187 = event-data() -> ()  [unwired: 1 in, 6 out]
            n188 = To Unsigned Byte Integer(number=w205) -> (unsigned 8bit integer=w204:u8)
            n189 = To Unsigned Byte Integer(number=w206) -> (unsigned 8bit integer=w203:u8)
            n190 = To Unsigned Byte Integer(number=w208) -> (unsigned 8bit integer=w207:u8)
            n191 = call "SendFLCam_DAC.vi"("ctrl"=w207, "feature"=w204, "data"="Offset ADC 1", "addr"=w203) -> ()
          }
          event "Offset ADC 6": Value Change {
            w212 = fxp<+,4,4> 0.0  # feature (hex)
            w213 = fxp<+,4,4> 3.0  # addr (hex)
            w215 = fxp<+,4,4> 3.0  # ctrl (hex)
            # "Register CHD"
            # "ctrl: write and update DAC register"
            n192 = event-data() -> ()  [unwired: 1 in, 6 out]
            n193 = To Unsigned Byte Integer(number=w212) -> (unsigned 8bit integer=w211:u8)
            n194 = To Unsigned Byte Integer(number=w213) -> (unsigned 8bit integer=w210:u8)
            n195 = To Unsigned Byte Integer(number=w215) -> (unsigned 8bit integer=w214:u8)
            n196 = call "SendFLCam_DAC.vi"("ctrl"=w214, "feature"=w211, "data"="Offset ADC 6", "addr"=w210) -> ()
          }
          event "Offset ADC 2": Value Change {
            w219 = fxp<+,4,4> 0.0  # feature (hex)
            w220 = fxp<+,4,4> 4.0  # addr (hex)
            w222 = fxp<+,4,4> 3.0  # ctrl (hex)
            # "Register CHE"
            # "ctrl: write and update DAC register"
            n197 = event-data() -> ()  [unwired: 1 in, 6 out]
            n198 = To Unsigned Byte Integer(number=w219) -> (unsigned 8bit integer=w218:u8)
            n199 = To Unsigned Byte Integer(number=w220) -> (unsigned 8bit integer=w217:u8)
            n200 = To Unsigned Byte Integer(number=w222) -> (unsigned 8bit integer=w221:u8)
            n201 = call "SendFLCam_DAC.vi"("ctrl"=w221, "feature"=w218, "data"="Offset ADC 2", "addr"=w217) -> ()
          }
          event "Offset ADC 7": Value Change {
            w226 = fxp<+,4,4> 0.0  # feature (hex)
            w227 = fxp<+,4,4> 5.0  # addr (hex)
            w229 = fxp<+,4,4> 3.0  # ctrl (hex)
            # "Register CHF"
            # "ctrl: write and update DAC register"
            n202 = event-data() -> ()  [unwired: 1 in, 6 out]
            n203 = To Unsigned Byte Integer(number=w226) -> (unsigned 8bit integer=w225:u8)
            n204 = To Unsigned Byte Integer(number=w227) -> (unsigned 8bit integer=w224:u8)
            n205 = To Unsigned Byte Integer(number=w229) -> (unsigned 8bit integer=w228:u8)
            n206 = call "SendFLCam_DAC.vi"("ctrl"=w228, "feature"=w225, "data"="Offset ADC 7", "addr"=w224) -> ()
          }
          event "Offset ADC 3": Value Change {
            w233 = fxp<+,4,4> 0.0  # feature (hex)
            w234 = fxp<+,4,4> 6.0  # addr (hex)
            w236 = fxp<+,4,4> 3.0  # ctrl (hex)
            # "Register CHG"
            # "ctrl: write and update DAC register"
            n207 = event-data() -> ()  [unwired: 1 in, 6 out]
            n208 = To Unsigned Byte Integer(number=w233) -> (unsigned 8bit integer=w232:u8)
            n209 = To Unsigned Byte Integer(number=w234) -> (unsigned 8bit integer=w231:u8)
            n210 = To Unsigned Byte Integer(number=w236) -> (unsigned 8bit integer=w235:u8)
            n211 = call "SendFLCam_DAC.vi"("ctrl"=w235, "feature"=w232, "data"="Offset ADC 3", "addr"=w231) -> ()
          }
          event "Offset ADC 8": Value Change {
            w240 = fxp<+,4,4> 0.0  # feature (hex)
            w241 = fxp<+,4,4> 7.0  # addr (hex)
            w243 = fxp<+,4,4> 3.0  # ctrl (hex)
            # "Register CHH"
            # "ctrl: write and update DAC register"
            n212 = event-data() -> ()  [unwired: 1 in, 6 out]
            n213 = To Unsigned Byte Integer(number=w240) -> (unsigned 8bit integer=w239:u8)
            n214 = To Unsigned Byte Integer(number=w241) -> (unsigned 8bit integer=w238:u8)
            n215 = To Unsigned Byte Integer(number=w243) -> (unsigned 8bit integer=w242:u8)
            n216 = call "SendFLCam_DAC.vi"("ctrl"=w242, "feature"=w239, "data"="Offset ADC 8", "addr"=w238) -> ()
          }
          event "send all": Value Change {
            n217 = event-data() -> ()  [unwired: 1 in, 6 out]
            n218 = property on="Offset ADC 4" class="DigNum (strict)"() -> ("Value"=w251:u16)  [unwired: 2 in, 2 out]
            n219 = property on="Offset ADC 6" class="DigNum (strict)"() -> ("Value"=w248:u16)  [unwired: 2 in, 2 out]
            n220 = property on="Offset ADC 5" class="DigNum (strict)"() -> ("Value"=w250:u16)  [unwired: 2 in, 2 out]
            n221 = property on="Offset ADC 1" class="DigNum (strict)"() -> ("Value"=w249:u16)  [unwired: 2 in, 2 out]
            n222 = property on="Offset ADC 4" class="DigNum (strict)"("Val(Sgnl)"=w251) -> ()  [unwired: 2 in, 2 out]
            n223 = property on="Offset ADC 6" class="DigNum (strict)"("Val(Sgnl)"=w248) -> ()  [unwired: 2 in, 2 out]
            n224 = property on="Offset ADC 5" class="DigNum (strict)"("Val(Sgnl)"=w250) -> ()  [unwired: 2 in, 2 out]
            n225 = property on="Offset ADC 1" class="DigNum (strict)"("Val(Sgnl)"=w249) -> ()  [unwired: 2 in, 2 out]
            n226 = property on="Offset ADC 8" class="DigNum (strict)"() -> ("Value"=w244:u16)  [unwired: 2 in, 2 out]
            n227 = property on="Offset ADC 2" class="DigNum (strict)"() -> ("Value"=w247:u16)  [unwired: 2 in, 2 out]
            n228 = property on="Offset ADC 3" class="DigNum (strict)"() -> ("Value"=w245:u16)  [unwired: 2 in, 2 out]
            n229 = property on="Offset ADC 7" class="DigNum (strict)"() -> ("Value"=w246:u16)  [unwired: 2 in, 2 out]
            n230 = property on="Offset ADC 8" class="DigNum (strict)"("Val(Sgnl)"=w244) -> ()  [unwired: 2 in, 2 out]
            n231 = property on="Offset ADC 2" class="DigNum (strict)"("Val(Sgnl)"=w247) -> ()  [unwired: 2 in, 2 out]
            n232 = property on="Offset ADC 3" class="DigNum (strict)"("Val(Sgnl)"=w245) -> ()  [unwired: 2 in, 2 out]
            n233 = property on="Offset ADC 7" class="DigNum (strict)"("Val(Sgnl)"=w246) -> ()  [unwired: 2 in, 2 out]
          }
        }
      }
    }
  }
  n234 = property on="sample" class="Slide (strict)"("DisabledEnum"=w1) -> ()  [unwired: 2 in, 2 out]
  n235 = property on="start" class="Bool (strict)"("DisabledEnum"=w1) -> ()  [unwired: 2 in, 2 out]
  n236 = property on="block" class="Slide (strict)"("DisabledEnum"=w1) -> ()  [unwired: 2 in, 2 out]
